vi "Impulse_response.vi"() -> ()   [LabVIEW 2018]
uses:
  <vilib>/DAQmx/read.llb/DAQmx Read (Analog 1D Wfm NChan NSamp).vi
  <vilib>/DAQmx/create/channels.llb/DAQmx Create Channel (AI-Acceleration-Accelerometer).vi
  <vilib>/DAQmx/configure/timing.llb/DAQmx Timing (Sample Clock).vi
  <vilib>/DAQmx/miscellaneous.llb/DAQmx Fill In Error Info.vi
  <resource>/objmgr/daqmx.rc
panel:
  out "error out":errorcluster
  out "Saving Data":bool
  out "Filename Out":path
  in  "Comment":string
  in  "Filename":path=path "test.lvm"
  in  "Enable":bool=TRUE
  in  "Reset":bool
  out "data":waveform(dbl)[](graph)
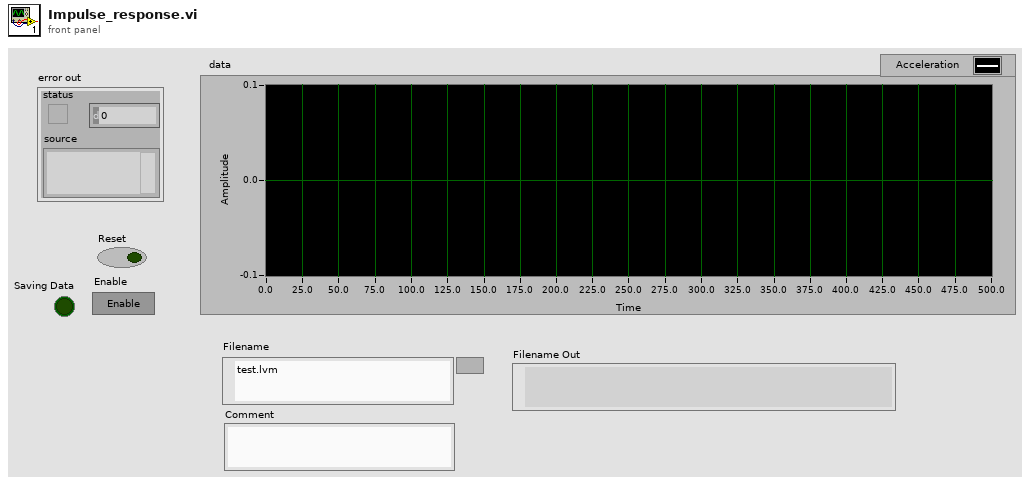
[diagram p1: front panel]
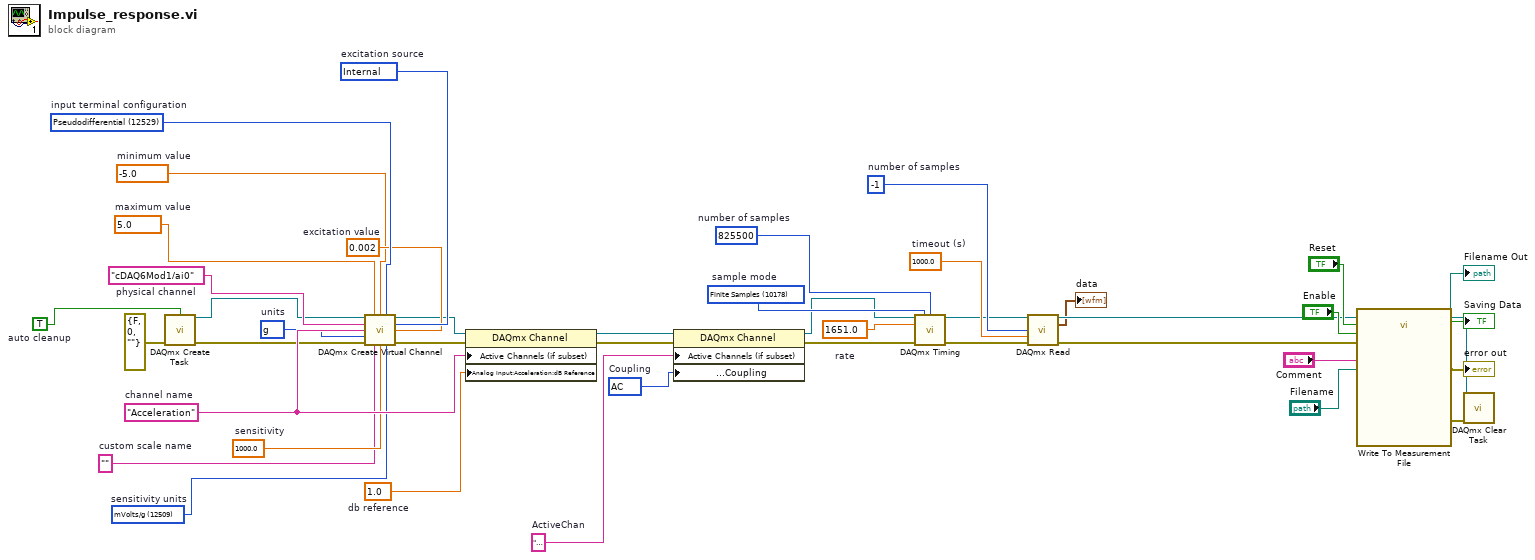
[diagram p0: block diagram]
diagram:
  w26 = 10178 items=["Finite Samples"=10178, "Continuous Samples"=10123, "Hardware Timed Single Point"=12522]  # sample mode
  w25 = 825500  # number of samples
  w24 = 1651.0  # rate
  w20 = 10045 items=["AC"=10045, "DC"=10050, "GND"=10066]  # Coupling
  w19 = "Acceleration"  # ActiveChan
  w17 = 1.0  # db reference
  w14 = 10186 items=["g"=10186, "m/s^2"=12470, "From Custom Scale"=10065]  # units
  w13 = 12529 items=["default"=-1, "RSE"=10083, "NRSE"=10078, "Differential"=10106, "Pseudodifferential"=12529]  # input terminal configuration
  w12 = 10200 items=["Internal"=10200, "External"=10167, "None"=10230]  # excitation source
  w11 = 0.002  # excitation value
  w10 = 12509 items=["mVolts/g"=12509, "Volts/g"=12510]  # sensitivity units
  w9 = 1000.0  # sensitivity
  w18 = "Acceleration"  # channel name
  w7 = ""  # custom scale name
  w6 = -5.0  # minimum value
  w5 = 5.0  # maximum value
  w4 = "cDAQ6Mod1/ai0"  # physical channel
  w2 = TRUE  # auto cleanup
  w34 = 1000.0  # timeout (s)
  w35 = -1  # number of samples
  n1 = call <vilib>:"DAQmx Create Task.vi"("auto cleanup"=w2, "error in"=errorcluster {"status"=FALSE, "code"=0, "source"=""}) -> ("task out"=w3:refnum<k21>, "error out"=w1:errorcluster)  [unwired: 12 in]
  n2 = call-poly <vilib>:"DAQmx Create Virtual Channel.vi"("task in"=w3, "maximum value"=w5, "minimum value"=w6, "input terminal configuration"=w13, "physical channels"=w4, "current excitation source"=w12, "name to assign"=w18, "current excitation value"=w11, "units"=w14, "error in"=w1, "custom scale name"=w7, "sensitivity"=w9, "sensitivity units"=w10) -> ("task out"=w8:refnum<k21>, "error out"=w15:errorcluster)  [unwired: 1 in]
  n3 = property class="DAQmx Channel"(reference=w8, error in=w15, "Active Channels (if subset)"=w18, "Analog Input:Acceleration:dB Reference"=w17) -> (reference out=w22:refnum<k21>, error out=w16:errorcluster)
  n4 = property class="DAQmx Channel"(reference=w22, error in=w16, "Active Channels (if subset)"=w19, "Analog Input:General Properties:Input Configuration:Coupling"=w20) -> (reference out=w23:refnum<k21>, error out=w21:errorcluster)
  n5 = call-poly <vilib>:"DAQmx Timing.vi"("task/channels in"=w23, "sample mode"=w26, "samples per channel"=w25, "rate"=w24, "error in"=w21) -> ("task out"=w32:refnum<k21>, "error out"=w31:errorcluster)  [unwired: 9 in]
  n6 = call-poly <vilib>:"DAQmx Read.vi"("task/channels in"=w32, "number of samples per channel"=w35, "timeout"=w34, "error in"=w31) -> ("task out"=w33:refnum<k21>, "data"=→"data":waveform(dbl)[], "error out"=w29:errorcluster)  [unwired: 9 in]
  n7 = call "Write To Measurement File"("Reset"="Reset", "Enable"="Enable", "error in (no error)"=w29, "Filename"="Filename", "Comment"="Comment") -> ("Filename Out"=→"Filename Out":path, "Saving Data"=→"Saving Data":bool, "error out"=w30:errorcluster)  [unwired: 12 in]
  "error out" <- w30
  n8 = call <vilib>:"DAQmx Clear Task.vi"("task in"=w33, "error in"=w30) -> ()  [unwired: 13 in, 1 out]
